vi "Zernike calc.vi"(0 "holo_init":u8[](array[numeric]), 5 "Zernike Coefs Cluster":T2 {"SecComaY" step=0.01; "SecComaX" step=0.01; "SecAstigY" step=0.01; "SecAstigX" step=0.01; "ComaY" step=0.01; "ComaX" step=0.01; "AstigY" step=0.01; "AstigX" step=0.01}, 9 "SLM Params":T1 {"Centre X" format="%.3g"; "Centre Y" format="%.3g"}, 11 "error in (no error)":errorcluster, 12 "radius":i32=1000) -> (4 "Zernike holo":u8[](array[numeric]), 15 "error out":errorcluster)   [LabVIEW 2020]
uses:
  _controls/PCIe SLM Zernike Coefs.ctl
  _controls/PCIe SLM params.ctl
  <userlib>/SLM ImageGen/SLM ImageGen.lvlib
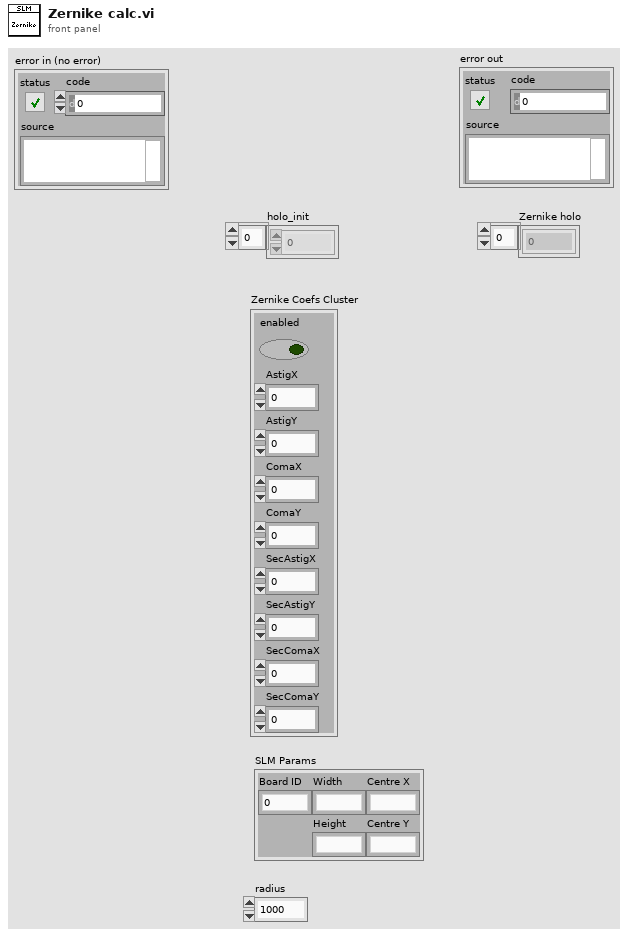
[diagram p1: front panel]
types:
  T1 = typedef "PCIe SLM params.ctl" = cluster{"Width":dbl, "Height":dbl, "Board ID":i32, "Centre Y":dbl, "Centre X":dbl}
  T2 = typedef "PCIe SLM Zernike Coefs.ctl" = cluster{"enabled":bool, "AstigX":dbl, "AstigY":dbl, "ComaX":dbl, "ComaY":dbl, "SecAstigX":dbl, "SecAstigY":dbl, "SecComaX":dbl, "SecComaY":dbl}
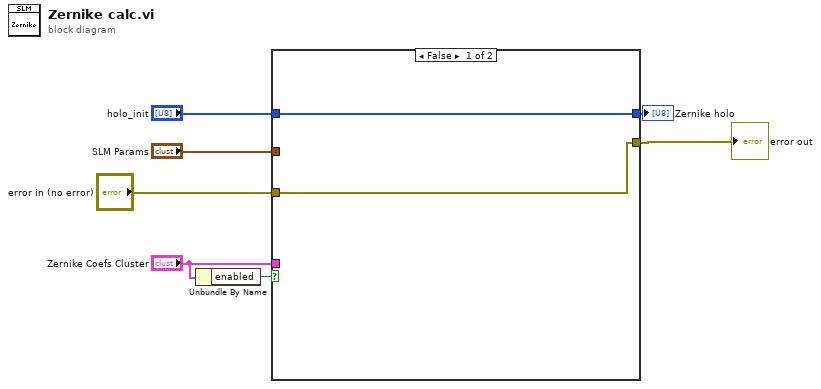
[diagram p0: block diagram]
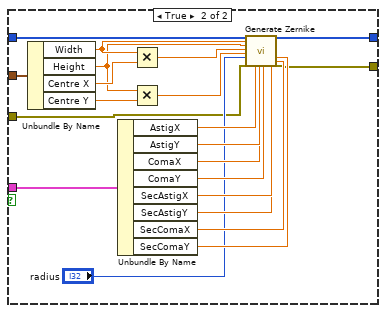
[diagram p2: hidden frame]
diagram:
  n1 = Unbundle By Name("Zernike Coefs Cluster") -> ("enabled"=w7:bool)
  n2 = case shown="False" w7 {
    tunnel: [w9 w19] -> w4
    tunnel: "holo_init" -> [w9 w30]
    tunnel: "Zernike Coefs Cluster" -> [_ w21]
    tunnel: "SLM Params" -> [_ w18]
    tunnel: [w8 w11] -> w2
    tunnel: "error in (no error)" -> [w8 w10]
    frame False {
    }
    frame True {
      n3 = Unbundle By Name(w18) -> ("Width"=w17:dbl, "Height"=w14:dbl, "Centre X"=w16:dbl, "Centre Y"=w13:dbl)
      n4 = Unbundle By Name(w21) -> ("AstigX"=w26:dbl, "AstigY"=w29:dbl, "ComaX"=w25:dbl, "ComaY"=w28:dbl, "SecAstigX"=w27:dbl, "SecAstigY"=w24:dbl, "SecComaX"=w23:dbl, "SecComaY"=w22:dbl)
      n5 = Multiply(x=w17, y=w16) -> (x*y=w15:dbl)
      n6 = Multiply(x=w14, y=w13) -> (x*y=w12:dbl)
      n7 = call <userlib>:"Generate Zernike.vi"("Array"=w30, "width"=w17, "height"=w14, "centerX"=w15, "centerY"=w12, "radius"="radius", "error in (no error)"=w10, "AstigX"=w26, "AstigY"=w29, "ComaX"=w25, "ComaY"=w28, "SecondaryAstigX"=w27, "SecondaryAstigY"=w24, "SecondaryComaY"=w22, "SecondaryComaX"=w23) -> ("Array out"=w19:u8[], "error out"=w11:errorcluster)  [unwired: 11 in]
    }
  }
  "Zernike holo" <- w4
  "error out" <- w2
